vi "BNO055 Write Reg.vi"(4 "Wait":u32, 6 "Data":u8[](array[numeric]) format="%.0x", 7 "Page":u8, 8 "error in (no error)":errorcluster, 9 "BNO055 Config Options":T1 {"ADC"."Comparator Queue & Disable" items=["Assert after one conversion", "Assert after two conversions", "Assert after four conversions", "Comparator disabled"]; "ADC"."Latching Comparator" items=["Non-latching", "Latching"]; "ADC"."Comparator Polarity" items=["Active Low", "Active High"]; "ADC"."Comparator Mode" items=["Traditional Comparator w/ hysteresis", "Window Comparator"]; "ADC"."Sampling Rate" items=["128SPS", "250SPS", "490SPS", "920SPS", "1600SPS", "2400SPS", "3300SPS"]; "ADC"."Sampling Mode" items=["Continuous Conversion", "Single-shot (Low Power)"]; "ADC"."Expected Range (Programmable Gain Amplifier)" items=["+/-6.144V", "+/-4.096V", "+/-2.048V", "+/-1.024V", "+/-0.512V", "+/-0.256V"]; "ADC"."Channel" items=["Differential: Ch 0&1", "Differential: Ch 0&3", "Differential: Ch 1&3", "Differential: Ch 2&3", "Single Ended: Ch 0", "Single Ended: Ch 1", "Single Ended: Ch 2", "Single Ended: Ch 3"]; "I2C"."Slave Address" format="%.0x"}, 10 "Register":u8 format="%.0x", 11 "LINX Resource in":T2) -> (0 "error out":errorcluster, 1 "BNO055 Config Options":T1 {"ADC"."Comparator Queue & Disable" items=["Assert after one conversion", "Assert after two conversions", "Assert after four conversions", "Comparator disabled"]; "ADC"."Latching Comparator" items=["Non-latching", "Latching"]; "ADC"."Comparator Polarity" items=["Active Low", "Active High"]; "ADC"."Comparator Mode" items=["Traditional Comparator w/ hysteresis", "Window Comparator"]; "ADC"."Sampling Rate" items=["128SPS", "250SPS", "490SPS", "920SPS", "1600SPS", "2400SPS", "3300SPS"]; "ADC"."Sampling Mode" items=["Continuous Conversion", "Single-shot (Low Power)"]; "ADC"."Expected Range (Programmable Gain Amplifier)" items=["+/-6.144V", "+/-4.096V", "+/-2.048V", "+/-1.024V", "+/-0.512V", "+/-0.256V"]; "ADC"."Channel" items=["Differential: Ch 0&1", "Differential: Ch 0&3", "Differential: Ch 1&3", "Differential: Ch 2&3", "Single Ended: Ch 0", "Single Ended: Ch 1", "Single Ended: Ch 2", "Single Ended: Ch 3"]; "I2C"."Slave Address" format="%.0x"}, 3 "LINX Resource out":T2)   [LabVIEW 2017]
uses:
  BNO055 Config Options.ctl
  <vilib>/MakerHub/LINX/Private/Type Defs/Platform.ctl
  <vilib>/MakerHub/LINX/Private/Type Defs/Interface.ctl
  <vilib>/MakerHub/LINX/Private/Device/Type Defs/TCP Config.ctl
  <vilib>/MakerHub/LINX/Private/Device/Type Defs/Channels.ctl
  <vilib>/MakerHub/LINX/Private/Device/Type Defs/LINX Device Config.ctl
  <vilib>/MakerHub/LINX/Private/Type Defs/LINX Ref.ctl
panel:
  # "NOT DONE\nYET!"
  # "NOT DONE\nYET!"
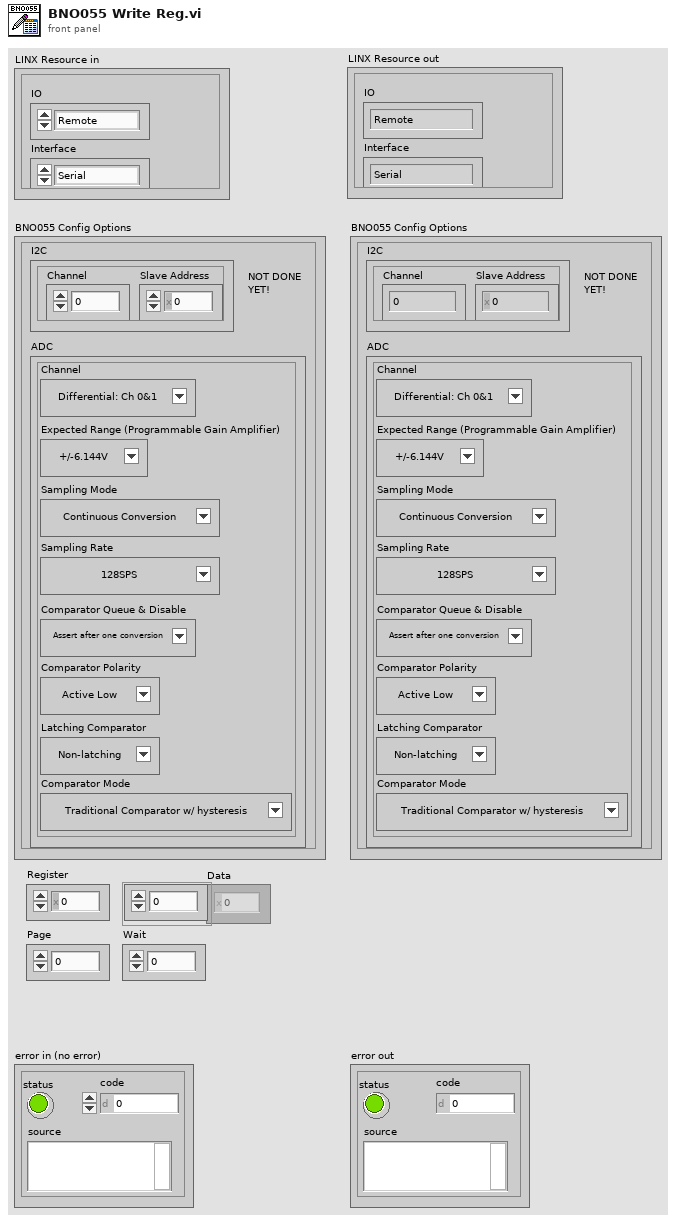
[diagram p1: front panel]
types:
  T1 = typedef "BNO055 Config Options.ctl" = cluster{"I2C":cluster{"Slave Address":u8, "Channel":u8}, "ADC":cluster{"Channel":u8, "Expected Range (Programmable Gain Amplifier)":u8, "Sampling Mode":u8, "Sampling Rate":u8, "Comparator Mode":u8, "Comparator Polarity":u8, "Latching Comparator":u8, "Comparator Queue & Disable":u8}}
  T2 = typedef "LMH-LINX.lvlib/LINX Ref.ctl" = cluster{"IO":T3, "Interface":T4, "LINX Device Config":T5}
  T3 = typedef "LMH-LINX.lvlib/Platform.ctl" = enum16{"Remote", "Local"}
  T4 = typedef "LMH-LINX.lvlib/Interface.ctl" = enum16{"Serial", "TCP"}
  T5 = typedef "LMH-LINX.lvlib/Device.lvlib/LINX Device Config.ctl" = cluster{"Interface":T4, "COM Port":refnum<visa-resource-name>, "TCP Configuration":T6, "Device Family":u8, "Device ID":u8, "Device Name":string, "TCP Ref":refnum<k5>, "Channels":T7}
  T6 = typedef "LMH-LINX.lvlib/Device.lvlib/TCP Config.ctl" = cluster{"IP Address":string, "Port":u16}
  T7 = typedef "LMH-LINX.lvlib/Channels.ctl" = cluster{"DI":u8[], "DO":u8[], "AI":u8[], "AO":u8[], "PWM":u8[], "QE":u8[], "UART":u8[], "I2C 2":u8[], "SPI":u8[], "CAN":u8[], "Servo":u8[], "AI Ref (V)":dbl, "AI Resolution (Bits)":u8, "AO Ref (V)":dbl, "AO Resolution (Bits)":u8}
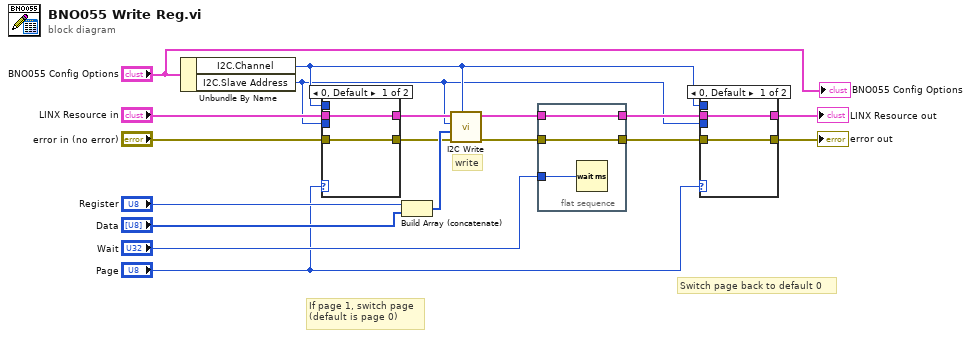
[diagram p0: block diagram]
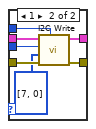
[diagram p2: hidden frame]
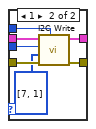
[diagram p3: hidden frame]
diagram:
  # "If page 1, switch page\n(default is page 0)"
  # "Switch page back to default 0"
  # "write"
  n1 = Unbundle By Name("BNO055 Config Options") -> ("I2C.Channel"=w9:u8, "I2C.Slave Address"=w7:u8)
  n2 = case shown="0, Default" "Page" {
    tunnel: "error in (no error)" -> [w19 w27]
    tunnel: "LINX Resource in" -> [w20 w26]
    tunnel: w7 -> [_ w25]
    tunnel: w9 -> [_ w24]
    tunnel: [w20 w23] -> w13
    tunnel: [w19 w22] -> w12
    frame 0, Default {
    }
    frame 1 {
      n3 = call <vilib>:"I2C Write.vi"("I2C Channel"=w24, "Error In"=w27, "Data"=u8[] [7, 1], "I2C Slave Address (0)"=w25, "LINX Resource"=w26) -> ("Error Out"=w22:errorcluster, "LINX Resource"=w23:T2)  [unwired: 5 in]
    }
  }
  n4 = Build Array (concatenate)("Register", "Data") -> (w14:u8[])
  n5 = call <vilib>:"I2C Write.vi"("I2C Channel"=w9, "Error In"=w12, "Data"=w14, "I2C Slave Address (0)"=w7, "LINX Resource"=w13) -> ("Error Out"=w11:errorcluster, "LINX Resource"=w10:T2)  [unwired: 5 in]
  n6 = flat-sequence {
    tunnel: [w30] -> w8
    tunnel: w10 -> [w30]
    tunnel: [w29] -> w6
    tunnel: w11 -> [w29]
    tunnel: "Wait" -> [w28]
    frame #0 {
      n7 = Wait (ms)(milliseconds to wait=w28) -> ()  [unwired: 1 out]
    }
  }
  n8 = case shown="0, Default" "Page" {
    tunnel: w6 -> [w31 w39]
    tunnel: w8 -> [w32 w38]
    tunnel: w7 -> [_ w37]
    tunnel: w9 -> [_ w36]
    tunnel: [w32 w35] -> w4
    tunnel: [w31 w34] -> w3
    frame 0, Default {
    }
    frame 1 {
      n9 = call <vilib>:"I2C Write.vi"("I2C Channel"=w36, "Error In"=w39, "Data"=u8[] [7, 0], "I2C Slave Address (0)"=w37, "LINX Resource"=w38) -> ("Error Out"=w34:errorcluster, "LINX Resource"=w35:T2)  [unwired: 5 in]
    }
  }
  "error out" <- w3
  "LINX Resource out" <- w4
  "BNO055 Config Options" <- "BNO055 Config Options"
